vi "example_LVUSBRH2_2.vi"() -> ()   [LabVIEW 2020]
uses:
  <vilib>/Instr/_visa.llb/VISA Flush IO Buffer Mask.ctl
  <vilib>/Instr/_visa.llb/VISA Configure Serial Port (Instr).vi
panel:
  in  "LED 2":bool
  in  "LED 1":bool
  in  "Btn stop":bool
  in  "VISA resource name":refnum<visa-resource-name>="COM1"
  # "Example 2: Turn On/Off LED1 or LED2 on USBRH2"
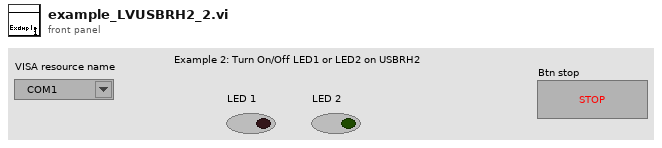
[diagram p1: front panel]
types:
  T1 = typedef "VISA Flush IO Buffer Mask.ctl" = u16
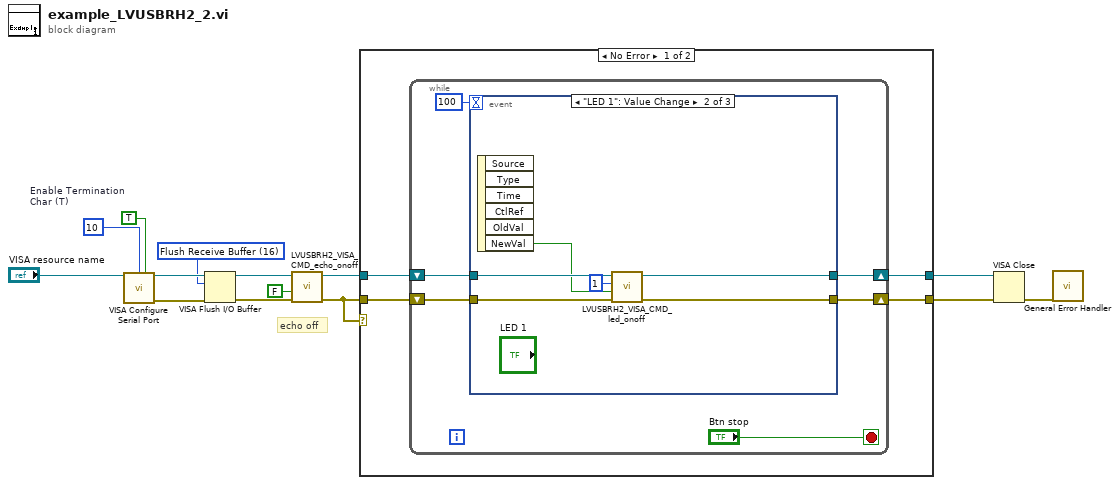
[diagram p0: block diagram]
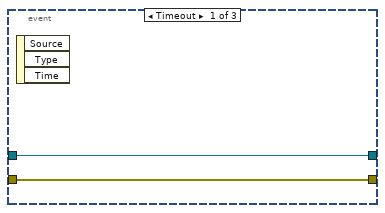
[diagram p2: hidden frame]
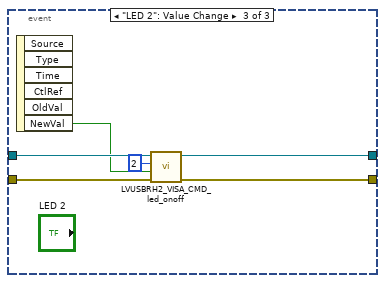
[diagram p3: hidden frame]
diagram:
  w1 = T1 16 items=["Flush Receive Buffer"=16, "Write Transmit Buffer to Device"=32, "Flush Receive Buffer (No I/O)"=64, "Flush Transmit Buffer"=128] ("Mask")
  w13 = TRUE  # Enable Termination Char (T)
  # "echo off"
  n1 = call-poly "VISA Configure Serial Port"("VISA resource name"="VISA resource name", "termination char\n(0xA = '\\n' = LF)"=u8 10 ("termination char\n(0xA = '\\n' = LF)"), "Enable Termination\nChar (T)"=w13) -> ("VISA resource name out"=w5:refnum<visa-resource-name>, "error out"=w4:errorcluster)  [unwired: 11 in]
  n2 = VISA Flush I/O Buffer(VISA resource name=w5, mask (16)=w1) -> (VISA resource name out=w6:refnum<visa-resource-name>)  [unwired: 1 in, 1 out]
  n3 = call "LVUSBRH2_VISA_CMD_echo_onoff.vi"("error in (no error)"=w4, "echo on/off)(F)"=FALSE, "VISA rssc"=w6) -> ("error out"=w2:errorcluster, "VISA rssc out"=w3:refnum<visa-resource-name>)  [unwired: 7 in]
  n4 = case shown="No Error" w2 {
    tunnel: w3 -> [w17 w39]
    tunnel: w2 -> [w16 w38]
    tunnel: [w15 w39] -> w11
    tunnel: [w14 w38] -> w10
    frame No Error {
      n5 = while {
        shift-right: [w19] -> w15
        shift-left: w17 -> [w21]
        shift-right: [w18] -> w14
        shift-left: w16 -> [w20]
        stop <- "Btn stop" stop-if-true
        n6 = event shown="[1] \"LED 1\": Value Change" {
          selector: _ -> [_ _ _]
          dyn-events: _ -> [_ _ _]
          timeout: 100 -> [_ _ _]
          tunnel: w21 -> [w25 w29 w35]
          tunnel: w20 -> [w24 w28 w34]
          tunnel: [w25 w30 w36] -> w19
          tunnel: [w24 w31 w37] -> w18
          event Timeout {
            n7 = event-data() -> ()  [unwired: 1 in, 3 out]
          }
          event "LED 1": Value Change {
            n8 = event-data() -> ("NewVal"=w27:bool)  [unwired: 1 in, 5 out]
            n9 = call "LVUSBRH2_VISA_CMD_led_onoff.vi"("error in (no error)"=w28, "Sw"=w27, "CH#(1)"=1, "VISA rssc"=w29) -> ("error out"=w31:errorcluster, "VISA rssc out"=w30:refnum<visa-resource-name>)  [unwired: 6 in]
          }
          event "LED 2": Value Change {
            n10 = event-data() -> ("NewVal"=w33:bool)  [unwired: 1 in, 5 out]
            n11 = call "LVUSBRH2_VISA_CMD_led_onoff.vi"("error in (no error)"=w34, "Sw"=w33, "CH#(1)"=2, "VISA rssc"=w35) -> ("error out"=w37:errorcluster, "VISA rssc out"=w36:refnum<visa-resource-name>)  [unwired: 6 in]
          }
        }
      }
    }
    frame Error {
    }
  }
  n12 = VISA Close(VISA resource name=w11, error in (no error)=w10) -> (error out=w8:errorcluster)
  n13 = call <vilib>:"General Error Handler.vi"("error in (no error)"=w8) -> ()  [unwired: 10 in, 5 out]
